vi "CopyGrayImg.vi"(1 "Image Name":string, 2 "Image In":T1) -> (0 "Image Out":T1)   [LabVIEW 2014]
uses:
  <vilib>/vision/Image Controls.llb/IMAQ Image.ctl
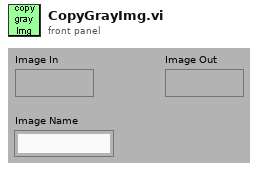
[diagram p1: front panel]
types:
  T1 = typedef "IMAQ Image.ctl" = refnum<image>
  T2 = typedef "Image Type" = u32
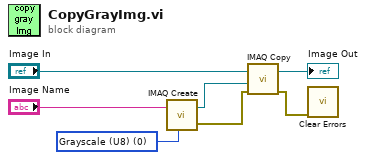
[diagram p0: block diagram]
diagram:
  w3 = T2 0 items=["Grayscale (U8)", "Grayscale (I16)", "Grayscale (SGL)", "Complex (CSG)", "RGB (U32)", "HSL (U32)", "RGB (U64)", "Grayscale (U16)"] ("Image Type")
  n1 = call "IMAQ Create"("Image Name"="Image Name", "Image Type"=w3) -> ("New Image"=w5:T1, "error out"=w2:errorcluster)  [unwired: 2 in, 1 out]
  n2 = call "IMAQ Copy"("error in (no error)"=w2, "Image Dst"=w5, "Image Src"="Image In") -> ("error out"=w1:errorcluster, "Image Dst Out"=→"Image Out":T1)  [unwired: 3 out]
  n3 = call <vilib>:"Clear Errors.vi"("error in (no error)"=w1) -> ()  [unwired: 5 in, 2 out]
